vi "Read Peaks.vi"(8 "error in (no error)":errorcluster, 11 "Spectrometer Driver in":refnum<class "Spectrometer Driver.lvclass">) -> (0 "error out":errorcluster, 2 "Peaks":T1={"Amplitude"=1000.0, "Center"=694.3, "Width"=0.4} {"Width" format="%#_gnm"; "Center" format="%#_gnm"}, 3 "Spectrometer Driver out":refnum<class "Spectrometer Driver.lvclass">)   [LabVIEW 2016, in "Spectrometer Driver.lvclass"]
uses:
  Spectrometer Driver.lvclass
  Utilities/Fit/Peak Parameters.ctl
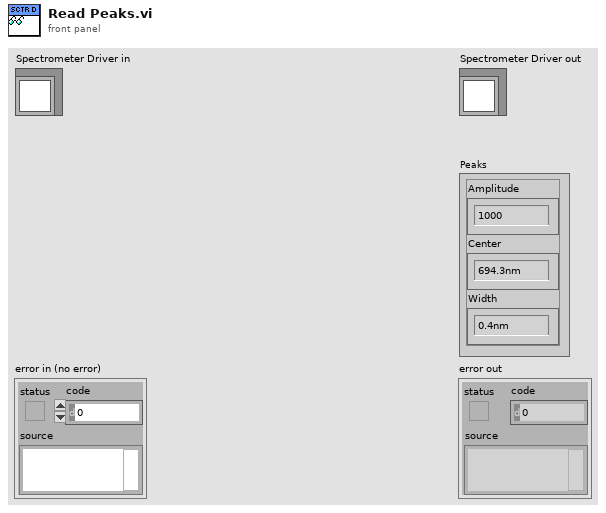
[diagram p1: front panel]
types:
  T1 = typedef "Peak Parameters.ctl" = cluster{"Amplitude":dbl, "Center":dbl, "Width":dbl}
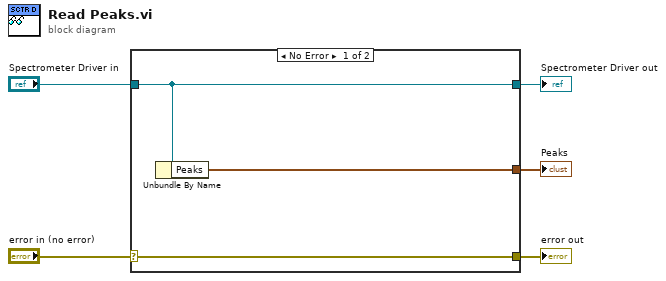
[diagram p0: block diagram]
diagram:
  n1 = case shown="No Error" "error in (no error)" {
    selector: "error in (no error)" -> [w8 w9]
    tunnel: [w8 w9] -> w4
    tunnel: [w7 w10] -> w2
    tunnel: "Spectrometer Driver in" -> [w7 w10]
    tunnel: [w6 _] -> w1
    frame No Error {
      n2 = Unbundle By Name(w7) -> ("Peaks"=w6:T1)
    }
    frame Error {
    }
  }
  "error out" <- w4
  "Spectrometer Driver out" <- w2
  "Peaks" <- w1
